vi "Save Configuration.vi"(5 "replace if found? (T)":bool=TRUE, 7 "create file if necessary (T)":bool=TRUE, 8 "error in (no error)":errorcluster, 9 "version (no change)":T1, 10 "Framework Configuration":refnum<class "Framework Configuration.lvclass">, 11 "configuration file path":path) -> (0 "error out":errorcluster, 3 "configuration file path dup":path, 4 "file replaced?":bool, 6 "file created?":bool)   [LabVIEW 2017, in "DSF Core.lvlib" / "Configuration Session.lvclass"]
doc: "Saves the provided <b>configuration</b> to the file located at the specified <b>configuration file path</b>."
uses:
  Configuration Session.lvclass
  Configuration/Framework/Framework Configuration.lvclass
  Typedefs/DSF Version Info.ctl
  DSF Core.lvlib
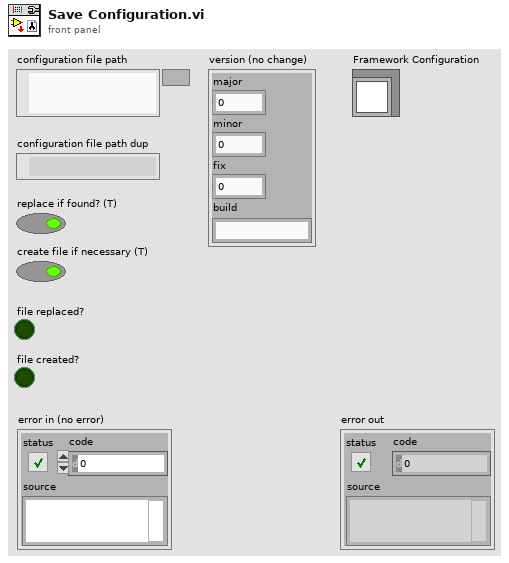
[diagram p1: front panel]
types:
  T1 = typedef "DSF Core.lvlib/DSF Version Info.ctl" = cluster{"major":u32, "minor":u32, "fix":u32, "build":string}
  T2 = typedef "DSF Core.lvlib/DSF Engine Framework Configuration.ctl" = cluster{"plugins":T3[]}
  T3 = typedef "DSF Core.lvlib/DSF Engine Plugin Configuration.ctl" = cluster{"core":T4, "component settings":T6[], "threads":T7[]}
  T4 = typedef "DSF Core.lvlib/DSF Core Plugin Configuration.ctl" = cluster{"name":string, "components":string[], "cycle timing":T5}
  T5 = typedef "DSF Core.lvlib/DSF Timing Info.ctl" = cluster{"priority":u64, "decimation":u64, "offset":u64}
  T6 = typedef "DSF Core.lvlib/DSF Settings Info.ctl" = cluster{"component":string, "version":T1, "values":cluster{"key":string, "value":string}[]}
  T7 = typedef "DSF Core.lvlib/DSF Engine Plugin Thread Configuration.ctl" = cluster{"core":T8, "component settings":T6[], "transfer groups":T9[]}
  T8 = typedef "DSF Core.lvlib/DSF Core Thread Configuration.ctl" = cluster{"processor":i32, "priority offset":i16}
  T9 = typedef "DSF Core.lvlib/DSF Engine Transfer Group Configuration.ctl" = cluster{"core":T10, "component settings":T6[], "transfers":T13[]}
  T10 = typedef "DSF Core.lvlib/DSF Core Group Configuration.ctl" = cluster{"name":string, "direction":T11, "cycle timing":T5, "timeout behavior":T12}
  T11 = typedef "DSF Core.lvlib/DSF Direction.ctl" = enum8{"Tx", "Rx"}
  T12 = typedef "DSF Core.lvlib/DSF Timeout Behavior.ctl" = enum8{"Increment Late Count", "Throw Error"}
  T13 = typedef "DSF Core.lvlib/DSF Engine Transfer Configuration.ctl" = cluster{"core":T14, "component settings":T6[], "channels":T15[]}
  T14 = typedef "DSF Core.lvlib/DSF Core Transfer Configuration.ctl" = cluster{"name":string}
  T15 = typedef "DSF Core.lvlib/DSF Engine Channel Configuration.ctl" = cluster{"core":T16, "component settings":T6[]}
  T16 = typedef "DSF Core.lvlib/DSF Core Channel Configuration.ctl" = cluster{"name":string, "units":string, "engine data type":T17, "string data type":T17, "string offset":u64}
  T17 = typedef "DSF Core.lvlib/DSF Data Type.ctl" = enum8{"Bool", "SGL", "DBL", "I8", "I16", "I32", "I64", "U8", "U16", "U32", "U64"}
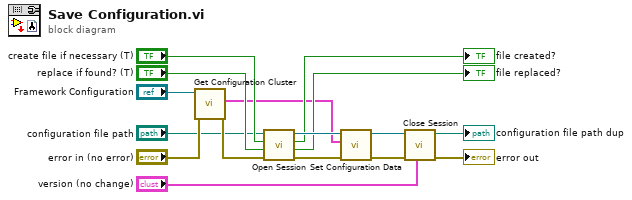
[diagram p0: block diagram]
diagram:
  n1 = call "Get Configuration Cluster.vi"("error in (no error)"="error in (no error)", "Framework Configuration in"="Framework Configuration") -> ("error out"=w2:errorcluster, "framework configuration"=w4:T2)  [unwired: 7 in, 1 out]
  n2 = call "Open Session.vi"("error in (no error)"=w2, "replace if found? (F)"="replace if found? (T)", "create file if necessary (T)"="create file if necessary (T)", "configuration file path"="configuration file path") -> ("error out"=w16:errorcluster, "file replaced?"=→"file replaced?":bool, "file created?"=→"file created?":bool, "configuration session"=w15:refnum<class "Configuration Session.lvclass">)  [unwired: 3 in, 1 out]
  n3 = call "Set Configuration Data.vi"("error in (no error)"=w16, "configuration data"=w4, "configuration session in"=w15) -> ("error out"=w14:errorcluster, "configuration session out"=w13:refnum<class "Configuration Session.lvclass">)  [unwired: 7 in]
  n4 = call "Close Session.vi"("version (no change)"="version (no change)", "error in (no error)"=w14, "configuration session"=w13) -> ("error out"=→"error out":errorcluster, "file path"=→"configuration file path dup":path)  [unwired: 7 in]
